vi "RichToFlatveristand_Request.vi"(5 "OutputClusterType":T1, 11 "InputCluster":T2) -> (3 "OutputCluster":T1)   [LabVIEW 2020, in "VeriStandgrpc_client.lvlib"]
uses:
  VeriStandgrpc_client.lvlib
  veristand_Request.ctl
  veristand_Request_Flat.ctl
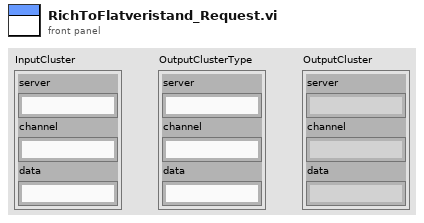
[diagram p1: front panel]
types:
  T1 = typedef "VeriStandgrpc_client.lvlib/veristand_Request_Flat.ctl" = cluster{"server":string, "channel":string, "data":string}
  T2 = typedef "VeriStandgrpc_client.lvlib/veristand_Request.ctl" = cluster{"server":string, "channel":string, "data":string}
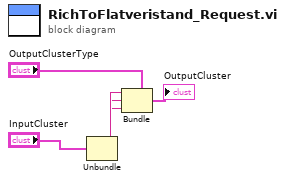
[diagram p0: block diagram]
diagram:
  n1 = Unbundle "Unbundle"("InputCluster") -> ("server"=w3:string, "channel"=w2:string, "data"=w1:string)
  n2 = Bundle "Bundle"(cluster="OutputClusterType", "server"=w3, "channel"=w2, "data"=w1) -> (→"OutputCluster":T1)
